vi "SVT Intermodulation Distortion.vi"   [LabVIEW 2017, in "SoundVib_Distortion.lvlib"]
doc: "Computes the total intermodulation distortion and the intermodulation components of <B>scaled signal [EU]</B> and <B>IMD standard</B>."
uses:
  <vilib>/addons/Sound and Vibration/svt_Distortion/SoundVib_Distortion.lvlib
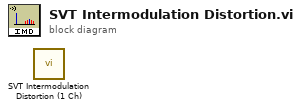
[diagram p0: block diagram]
diagram:
  n1 = call <vilib>:"SVT Intermodulation Distortion (1 Ch).vi"() -> ()  [unwired: 12 in, 8 out]
